vi "Update DaqLoopTimer Q.vi"(6 "elapsed time (ms)":u32, 7 "AI TaskName":string) -> ()   [LabVIEW 2017, in "DAQ.lvclass"]
doc: "Developed by Kevin Thompson\nThompson Engineering, LLC\nkevin@thompsonengineering.net"
uses:
  DAQ.lvclass
  TD DaqLoopTime DataQ--ref.ctl
  GBL DataQ Refs.vi
panel:
  out "DaqData ElapsedTimeRef":T1
  out "error out":errorcluster
  in  "error in (no error)":errorcluster
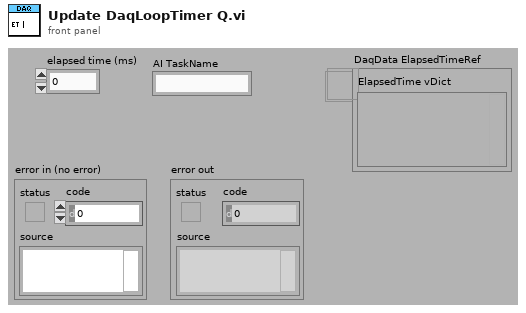
[diagram p1: front panel]
types:
  T1 = typedef "DAQ.lvclass/TD DaqLoopTime DataQ--ref.ctl" = refnum<queue>
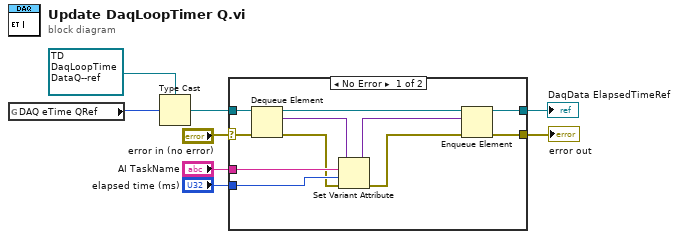
[diagram p0: block diagram]
diagram:
  n1 = global read "GBL DataQ Refs.vi" "DAQ eTime QRef"() -> (w3:u32)
  n2 = Type Cast(type=T1 refnum ("DaqData ElapsedTimeRef"), x=w3) -> (*(type *) &x=w1:T1)
  n3 = case shown="No Error" "error in (no error)" {
    selector: "error in (no error)" -> [w15 w20]
    tunnel: w1 -> [w19 w21]
    tunnel: [w17 w20] -> w7
    tunnel: [w16 w21] -> w8
    tunnel: "AI TaskName" -> [w14 _]
    tunnel: "elapsed time (ms)" -> [w13 _]
    frame No Error {
      n4 = Dequeue Element(queue=w19, error in (no error)=w15) -> (queue out=w18:T1, element=w12:variant, error out=w10:errorcluster)  [unwired: 1 in, 1 out]
      n5 = Set Variant Attribute(Variant=w12, name=w14, value=w13, error in=w10) -> (Variant out=w11:variant, error out=w9:errorcluster)  [unwired: 1 out]
      n6 = Enqueue Element(queue=w18, element=w11, error in (no error)=w9) -> (queue out=w16:T1, error out=w17:errorcluster)  [unwired: 1 in, 1 out]
    }
    frame Error {
    }
  }
  "error out" <- w7
  "DaqData ElapsedTimeRef" <- w8
